vi "GreekCode.vi"(1 "Number":u64=1 min=1 max=8308824) -> (0 "Result":string)   [LabVIEW 2014]
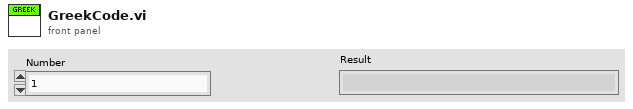
[diagram p1: front panel]
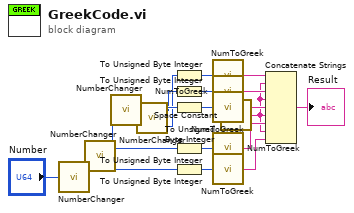
[diagram p0: block diagram]
diagram:
  n1 = call "NumberChanger.vi"("Input"="Number") -> ("New Value"=w17:u64, "Value 2"=w20:u64)
  n2 = call "NumberChanger.vi"("Input"=w20) -> ("New Value"=w11:u64, "Value 2"=w19:u64)
  n3 = call "NumberChanger.vi"("Input"=w19) -> ("New Value"=w10:u64, "Value 2"=w18:u64)
  n4 = call "NumberChanger.vi"("Input"=w18) -> ("New Value"=w9:u64, "Value 2"=w8:u64)
  n5 = To Unsigned Byte Integer(number=w8) -> (unsigned 8bit integer=w12:u8)
  n6 = To Unsigned Byte Integer(number=w9) -> (unsigned 8bit integer=w13:u8)
  n7 = To Unsigned Byte Integer(number=w10) -> (unsigned 8bit integer=w14:u8)
  n8 = To Unsigned Byte Integer(number=w11) -> (unsigned 8bit integer=w15:u8)
  n9 = To Unsigned Byte Integer(number=w17) -> (unsigned 8bit integer=w16:u8)
  n10 = call "NumToGreek.vi"("Number"=w12) -> ("Greek Letter"=w7:string)
  n11 = call "NumToGreek.vi"("Number"=w13) -> ("Greek Letter"=w6:string)
  n12 = call "NumToGreek.vi"("Number"=w14) -> ("Greek Letter"=w5:string)
  n13 = call "NumToGreek.vi"("Number"=w15) -> ("Greek Letter"=w4:string)
  n14 = call "NumToGreek.vi"("Number"=w16) -> ("Greek Letter"=w2:string)
  n15 = call <vilib>:"Space Constant.vi"() -> ("String"=w3:string)
  n16 = Concatenate Strings(w7, w3, w6, w3, w5, w3, w4, w3, w2) -> (→"Result":string)
